vi "Send Get Connection List.vi"(7 "Priority":T1=enum."Normal" caption="Message Priority (Normal)", 8 "error in (no error)":errorcluster, 11 "Message Enqueuer in":refnum<class "Message Enqueuer.lvclass">) -> (0 "error out":errorcluster, 2 "Connection List":refnum<class "Message Enqueuer.lvclass">[](array[class]), 3 "Message Enqueuer out":refnum<class "Message Enqueuer.lvclass">)   [LabVIEW 2017, in "Connection Listener.lvlib" / "Get Connection List Msg.lvclass"]
doc: "Sends the <b>Connection Listener.lvlib:Get Connection List Msg.lvclass</b> message.\n\nThis message will call <b>Get Connection List.vi</b> on the <b>Connection Listener.lvlib:Connection Listener.lvclass</b> actor.\n\n<b>Get Connection List.vi Description</b>"
uses:
  Get Connection List Msg.lvclass
  <vilib>/ActorFramework/Message Enqueuer/Message Enqueuer.lvclass
  <vilib>/ActorFramework/Message Enqueuer/Message Priority.ctl
  Applications/National Instruments/LabVIEW 2017 64-bit/vi.lib/ActorFramework/Reply Msg/Reply Msg.lvclass
  <vilib>/ActorFramework/Reply Msg/Reply Msg.lvclass/Reply Msg.ctl
  <vilib>/ActorFramework/Message Enqueuer/Message Enqueuer.lvclass/Message Enqueuer.ctl
  <vilib>/ActorFramework/Message Enqueuer/Enqueue.vi
  <vilib>/ActorFramework/Reply Msg/Reply Msg.lvclass
  Applications/National Instruments/LabVIEW 2017 64-bit/vi.lib/ActorFramework/Message/Message.lvclass
  <vilib>/ActorFramework/Message Priority Queue/Priority Enqueue.vi
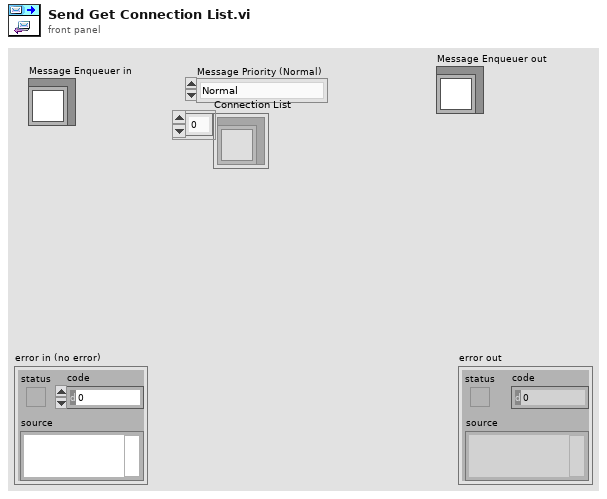
[diagram p1: front panel]
types:
  T1 = typedef "Actor Framework.lvlib/Message Enqueuer.lvclass/Message Priority.ctl" = enum16{"Low", "Normal", "High"}
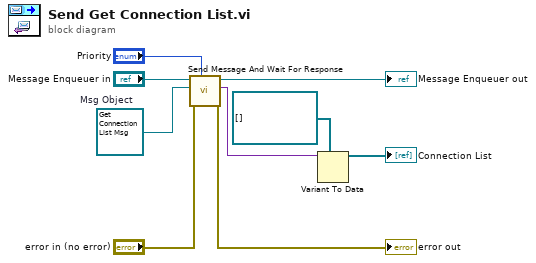
[diagram p0: block diagram]
diagram:
  w5 = refnum<class "Get Connection List Msg.lvclass"> refnum  # Msg Object
  n1 = call <vilib>:"Send Message And Wait For Response.vi"("Message Priority (Normal)"="Priority", "error in (no error)"="error in (no error)", "Original Message"=w5, "Message Enqueuer in"="Message Enqueuer in") -> ("error out"=→"error out":errorcluster, "Reply"=w3:variant, "Message Enqueuer out"=→"Message Enqueuer out":refnum<class "Message Enqueuer.lvclass">)  [unwired: 4 in, 1 out]
  n2 = Variant To Data(type=refnum<class "Message Enqueuer.lvclass">[] [] ("ConnHandlers"), Variant=w3) -> (data=→"Connection List":refnum<class "Message Enqueuer.lvclass">[])  [unwired: 1 in, 1 out]
